vi "Logging Active.vi"(8 "error in (no error)":errorcluster, 11 "State Machine in":refnum<class "State Machine.lvclass">) -> (0 "error out":errorcluster, 3 "State Machine out":refnum<class "State Machine.lvclass">)   [LabVIEW 2024, in "State Machine.lvlib" / "State Machine.lvclass"]
uses:
  State Machine.lvclass
  State Machine.lvclass/State Machine.ctl
  State/State/State.lvclass
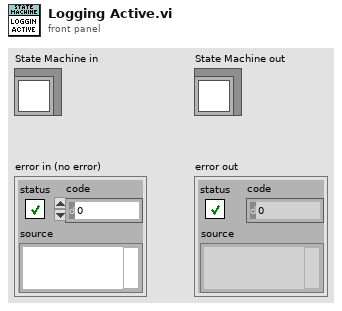
[diagram p1: front panel]
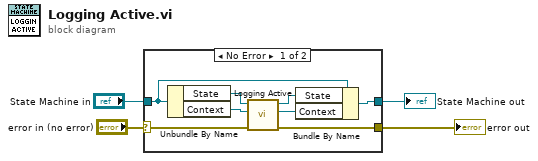
[diagram p0: block diagram]
diagram:
  n1 = case shown="No Error" "error in (no error)" {
    selector: "error in (no error)" -> [w6 w14]
    tunnel: [w5 w14] -> w3
    tunnel: [w11 w13] -> w1
    tunnel: "State Machine in" -> [w12 w13]
    frame No Error {
      n2 = Unbundle By Name(w12) -> ("State"=w10:refnum<class "State.lvclass">, "Context"=w9:refnum<class "Context.lvclass">)
      n3 = call-dynamic "Logging Active.vi"("error in (no error)"=w6, "Context in"=w9, "State in"=w10) -> ("error out"=w5:errorcluster, "Context out"=w7:refnum<class "Context.lvclass">, "State out"=w8:refnum<class "State.lvclass">)  [unwired: 6 in]
      n4 = Bundle By Name(cluster=w12, "State"=w8, "Context"=w7) -> (w11:refnum<class "State Machine.lvclass">)
    }
    frame Error {
    }
  }
  "error out" <- w3
  "State Machine out" <- w1
